vi "set Disappearing.vi"(10 "Disappearing":bool, 11 "Element in":refnum<class "Element.lvclass">) -> (3 "Element out":refnum<class "Element.lvclass">)   [LabVIEW 2021, in "Element.lvclass"]
uses:
  Element.lvclass
  Element.lvclass/Element.ctl
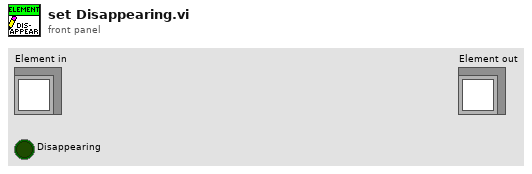
[diagram p1: front panel]
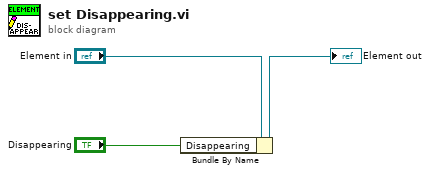
[diagram p0: block diagram]
diagram:
  n1 = Bundle By Name(cluster="Element in", "Disappearing"="Disappearing") -> (→"Element out":refnum<class "Element.lvclass">)
